vi "PathConfiguration.vi"() -> ()   [LabVIEW 2017]
panel:
  in  "Top Level Output Path":path
  in  "Output Path":path
  in  "Input Path":path
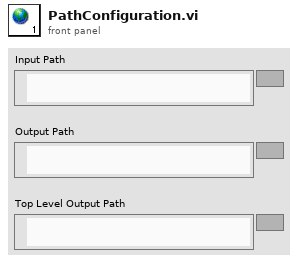
[diagram p1: front panel]
diagram:
